vi "AlliGator Run XY Graph Python Function (API v1.1).vi"(6 "Mouse Click Event Data":T1, 7 "AlliGator Ctrl Refnums":T8, 8 "error in (no error)":errorcluster, 9 "data value reference in":refnum<data-value>, 10 "Python Function Info":T4, 11 "Python Session ID":refnum<k35>) -> (0 "error out":errorcluster, 1 "Data Value Reference out":refnum<data-value>, 2 "JSON String":string, 3 "Function Display Name":string, 4 "Function Parameters JSON String":string, 5 "Message":string)   [LabVIEW 2021, in "AlliGator Python Plugins.lvlib"]
uses:
  AlliGator Python Plugins.lvlib
  GUI/AlliGator Ctrl Refnums.ctl
  GUI/AlliGator Other Ctrl Refnums.ctl
  GUI/AlliGator State Indicator.ctl
  GUI/AlliGator Main Window Tabs.ctl
  GUI/AlliGator Phasor Plot Ctrl Refnums.ctl
  GUI/AlliGator Phasor Graph Ctrl Refnums.ctl
  Phasor/Phasor Calibration Type.ctl
  GUI/AlliGator Dataset Ctrl Refnums.ctl
  Source Image/AlliGator Displayed Image.ctl
  GUI/AlliGator Registered Events Ctrl Refnums.ctl
  GUI/AlliGator Image Histogram Control Refnums.ctl
  Histograms/Linear Histogram Options.ctl
  Histograms/Histogram Bin Option.ctl
  Histograms/Histogram Bin Position.ctl
  Decay Fit Parameter Map/AlliGator Decay Fit Map Control Refnums.ctl
  Fits/IRF(X)PSED/Decay Fit Parameters & Derived Quantities List v2.ctl
  Parameter Map/AlliGator Parameter Map Control Refnums.ctl
  Internal Variables/AlliGator Internal Variables v2.ctl
  <vilib>/vision/Image Controls.llb/IMAQ Image.ctl
  Internal Variables/AlliGator Gate Image Set.ctl
  Files/AlliGator FLI Dataset Type.ctl
  Files/AlliGator Data Series Type.ctl
  Dual-Channel Datasets/AlliGator Dataset Channel.ctl
  Settings/AlliGator Gate Arithmetic.ctl
  Image/Named ROI Description.ctl
  Phasor Graph/AlliGator Decay Metadata v3.ctl
  Decay Analysis/Decay Preprocessing/AlliGator Decay Background Subtraction Info.ctl
  Decay Analysis/Decay Preprocessing/AlliGator Baseline Subtraction Method.ctl
  Graphs/XY Graph/XY Graph Plot Shift Parameters.ctl
  Graphs/XY Graph/XY Graph Plot Shift Method.ctl
  Decay Analysis/Decay Preprocessing/AlliGator Decay Extrapolation Parameters.ctl
  Phasor/Calibration Phasor (m, phi).ctl
  Phasor/Phasor Reference Series.ctl
  Phasor/Phasor Calibration Map v2.ctl
  Phasor/Phasor (g, s).ctl
  Phasor Graph/AlliGator Raw Phasor Plot Data v5.ctl
  Phasor/Phasor Standard Deviation Options.ctl
  Phasor Plot/AlliGator Phasor Multi-Harmonic Data.ctl
  Phasor/Phasor Harmonic Data.ctl
  Decay Fit Parameter Map/AlliGator Decay Fit Options & Parameters v4.ctl
  Fits/IRF(X)PSED/Decay Fit Options v4.ctl
  Fits/Decay Convolution/Decay Model.ctl
  Fits/Residual Type.ctl
  Fits/IRF(X)PSED/Fit Weights Type v2.ctl
  Fits/Non-linear Fitting Method v2.ctl
  Fits/Fit Calculation Method.ctl
  Fits/Non-linear Fitting Algorithm.ctl
  Decay Analysis/Decay Fit/AlliGator Decay Fit Parameter Constraints 2.ctl
  Fits/IRF(X)PSED/Decay Fit Parameters In List.ctl
  Fits/IRF(X)PSED/MLE Baseline Offset Type.ctl
  Decay Analysis/Decay Preprocessing/AlliGator Decay Preprocessing Parameters.ctl
  Fits/IRF(X)PSED/Decay Fit Result Constraint.ctl
  Decay Fit Parameter Map/AlliGator Parameter Maps Data.ctl
  AlliGator Python Function Information.ctl
  AlliGator Python Function Parameter Definition.ctl
  AlliGator Python Function Output Definition.ctl
  AlliGator Python Plugin Target Type.ctl
  Graphs/XY Graph/XY Graph Mouse Click Event Data.ctl
  Graphs/XY Graph/XY Graph Refnum.ctl
  <vilib>/Utility/miscctls.llb/LVPoint32TypeDef.ctl
  API v1/AlliGator Python Plugin Plot Data v1.ctl
  API v1/AlliGator Python Plugin Graph Data v1.ctl
  AlliGator Python Plugin Data v1.1.ctl
  API v1/AlliGator Python Plugin Image Data v1.ctl
  AlliGator Python Plugin Parameter Map Data v1.1.ctl
  Image/Image Point.ctl
  AlliGator Python Plugin FLI Dataset Data v1.1.ctl
  Graphs/Get Plot at Mouse Click (XY Graph)/Get Plot at Mouse Click [AAC].vi
  Graphs/Graphs.lvlib
  Graphs/XY Graph/XY Graph Add-Ons.lvlib
  Strings/Strings.lvlib
  Error/Error.lvlib
  Image/Image.lvlib
  GUI/AlliGator GUI.lvlib
  Source Image/AlliGator Source Image.lvlib
  Phasor/Phasor.lvlib
  Histograms/Histogram Window.lvlib
  Fits/Fits.lvlib
  Decay Fit Parameter Map/AlliGator Decay Fit Parameter Map.lvlib
  Parameter Map/AlliGator Parameter Map.lvlib
  Decay Analysis/Decay Preprocessing/AlliGator Decay Preprocessing.lvlib
  Phasor Graph/AlliGator Phasor Graph.lvlib
  Files/AlliGator Files.lvlib
  Internal Variables/AlliGator Internal Variables.lvlib
  Phasor Plot/AlliGator Phasor Plot.lvlib
  Decay Analysis/Decay Fit/AlliGator Decay Fit.lvlib
  Settings/AlliGator Settings.lvlib
  Dual-Channel Datasets/AlliGator Dual-Channel Datasets.lvlib
panel:
  # "see the License on the block diagram (Ctrl+E or Window:Show Block Diagram)"
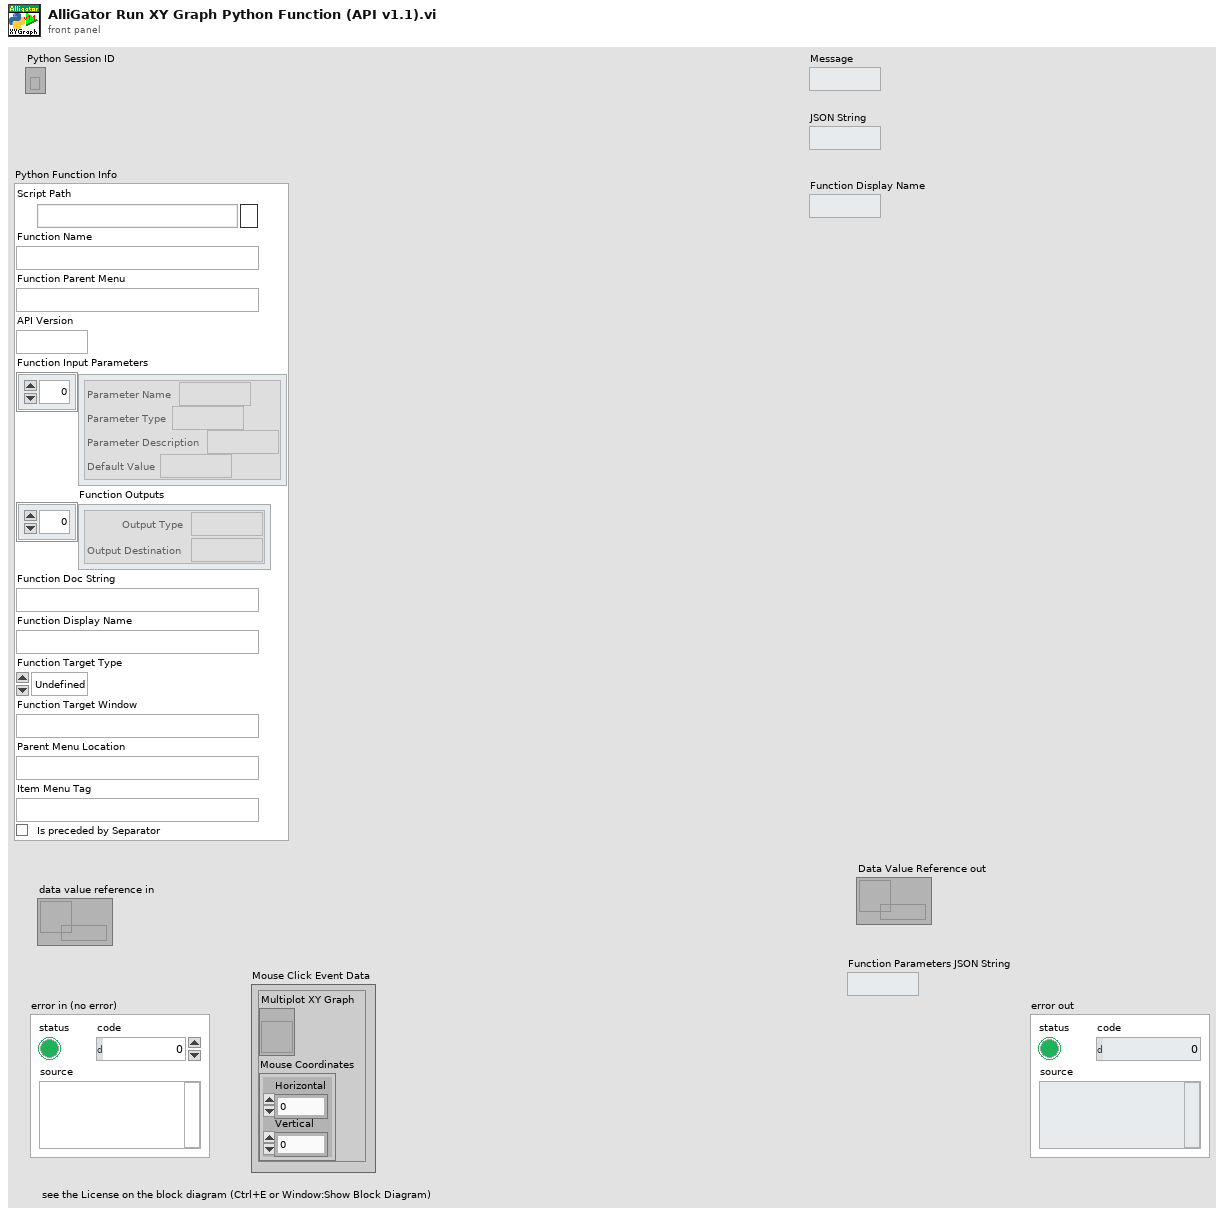
[diagram p1: front panel]
types:
  T1 = typedef "XY Graph Add-Ons.lvlib/XY Graph Mouse Click Event Data.ctl" = cluster{"Multiplot XY Graph":T2, "Mouse Coordinates":T3}
  T2 = typedef "XY Graph Add-Ons.lvlib/XY Graph Refnum.ctl" = refnum<vi>
  T3 = typedef "LVPoint32TypeDef.ctl" = cluster{"Horizontal":i32, "Vertical":i32}
  T4 = typedef "AlliGator Python Plugins.lvlib/AlliGator Python Function Information.ctl" = cluster{"Script Path":path, "Function Name":string, "Function Parent Menu":string, "API Version":string, "Function Input Parameters":T5[], "Function Outputs":T6[], "Function Doc String":string, "Function Display Name":string, "Function Target Type":T7, "Function Target Window":string, "Parent Menu Location":string, "Item Menu Tag":string, "Is preceded by Separator":bool}
  T5 = typedef "AlliGator Python Plugins.lvlib/AlliGator Python Function Parameter Definition.ctl" = cluster{"Parameter Name":string, "Parameter Type":string, "Parameter Description":string, "Default Value":string}
  T6 = typedef "AlliGator Python Plugins.lvlib/AlliGator Python Function Output Definition.ctl" = cluster{"Output Type":string, "Output Destination":string}
  T7 = typedef "AlliGator Python Plugins.lvlib/AlliGator Python Plugin Target Type.ctl" = enum16{"Undefined", "Window Menu", "Object Menu"}
  T8 = typedef "AlliGator GUI.lvlib/AlliGator Ctrl Refnums.ctl" = cluster{"Other AlliGator Ctrl Refnums":T9, "Phasor Plot Ctrl Refnums":T10, "Phasor Graph Ctrl Refnums":T11, "Dataset Control Refnums":T12, "Registered Events Ctrl Refnums":T13, "Image Histogram Ctrl Refnums":T14, "Decay Fit Map Ctrl Refnums":T15, "Parameter Map Ctrl Refnums":T16}
  T9 = typedef "AlliGator GUI.lvlib/AlliGator Other Ctrl Refnums.ctl" = cluster{"State Indicators":refnum<vi>, " Progress Bar":refnum<vi>, "Decay Graph Active":refnum<vi>, "Decay Statistics Bin":refnum<vi>, "Time Step":refnum<vi>, "Use File Timestamp":refnum<vi>, "Tab Control":refnum<vi>, "CPU":refnum<vi>, "Abort Fit":refnum<vi>, "Dataset File/Folder Path":refnum<vi>, "Abort ROI Creation":refnum<vi>, "Event LED":refnum<vi>, "Dataset File/Folder Path 2":refnum<vi>, "Dataset File/Folder Path 3":refnum<vi>, "Dataset File/Folder Path 4":refnum<vi>, "Dataset File/Folder Path 5":refnum<vi>, "Dataset File/Folder Path 6":refnum<vi>, "Dataset File/Folder Path 7":refnum<vi>, "Dataset File/Folder Path 8":refnum<vi>, "Dataset File/Folder Path 9":refnum<vi>, "Dataset File/Folder Path 10":refnum<vi>, "Dataset File/Folder Path 11":refnum<vi>}
  T10 = typedef "AlliGator GUI.lvlib/AlliGator Phasor Plot Ctrl Refnums.ctl" = cluster{"Phasor Ratio":refnum<vi>, "Modulus Lifetime":refnum<vi>, "Phasor at cursor (m, phi)":refnum<vi>, "Phase Lifetime":refnum<vi>, "Phasor at cursor (g, s)":refnum<vi>, "Phasor Plor Average Lifetime":refnum<vi>, "Phasor Plot Active":refnum<vi>, "Save Phasor Plot":refnum<vi>, "Image Overlay Color":refnum<vi>, "Phasor Plot Color Scale":refnum<vi>, "Reference 1 Button":refnum<vi>, "Reference 2 Button":refnum<vi>, "True Phasor Plot Value":refnum<vi>}
  T11 = typedef "AlliGator GUI.lvlib/AlliGator Phasor Graph Ctrl Refnums.ctl" = cluster{"Phasor Ratio":refnum<vi>, "Modulus Lifetime":refnum<vi>, "Phasor at cursor (m, phi)":refnum<vi>, "Phase Lifetime":refnum<vi>, "Phasor at cursor (g, s)":refnum<vi>, "Phasor Graph Average Lifetime":refnum<vi>, "Phasor Graph Active":refnum<vi>, "Save Phasor Graph":refnum<vi>, "Phasor Frame Slide":refnum<vi>, "Single Step Phasor":refnum<vi>, "Calibration Type":refnum<vi>, "Show Line":refnum<vi>, "Phase Lifetime 1":refnum<vi>, "Phase Lifetime 2":refnum<vi>, "Phasor Graph Frequency":refnum<vi>, "Phasor Reference 1 Control":refnum<vi>, "Phasor Reference 2 Control":refnum<vi>, "Calibration Lifetime":refnum<vi>, "Phase Lifetime SDV":refnum<vi>, "Average Lifetime SDV":refnum<vi>, "Phasor Ratio SDV":refnum<vi>, "Modulus Lifetime SDV":refnum<vi>}
  T12 = typedef "AlliGator GUI.lvlib/AlliGator Dataset Ctrl Refnums.ctl" = cluster{"Current Data":refnum<vi>, "Gate Image Slide":refnum<vi>, "Time Point Slide":refnum<vi>, "Current Time Stamp":refnum<vi>, "Save Image":refnum<vi>, "Displayed Image":refnum<vi>, "Overlay Mode":refnum<vi>, "Phasor Overlay Color":refnum<vi>, "Image Color Scale":refnum<vi>, "Use ROI as Search Area":refnum<vi>, "Source Image ROI Color":refnum<vi>, "True Pixel Value":refnum<vi>}
  T13 = typedef "AlliGator GUI.lvlib/AlliGator Registered Events Ctrl Refnums.ctl" = cluster{"Time Point Slider":refnum<vi>, "Phasor Plot Display Range":refnum<vi>, "Decay Graph":refnum<vi>, "Decay Statistics Graph":refnum<vi>, "Intensity Time Trace":refnum<vi>, "Phasor Graph":refnum<vi>, "Phasor Ratio Graph":refnum<vi>, "Lifetime Graph":refnum<vi>, "Phasor Plot Display":refnum<vi>, "Source Image Display":refnum<vi>, "Decay Fit Parameter Map Display Range":refnum<vi>, "Decay Fit Parameter Map Display":refnum<vi>, "Parameter Map Display Range":refnum<vi>, "Parameter Map Display":refnum<vi>, "Phasor Plot Display Range":refnum<vi>}
  T14 = typedef "AlliGator GUI.lvlib/AlliGator Image Histogram Control Refnums.ctl" = cluster{"Image Histogram":refnum<vi>, "Image Histogram Options":refnum<vi>, "Image Histogram Active":refnum<vi>, "Image Histogram Upper Percentile":refnum<vi>, "Image Histogram Lower Percentile":refnum<vi>, "Auto-Adjust Contrast":refnum<vi>}
  T15 = typedef "AlliGator Decay Fit Parameter Map.lvlib/AlliGator Decay Fit Map Control Refnums.ctl" = cluster{"Decay Fit Parameter Map Color Scale":refnum<vi>, "Decay Fit Parameter":refnum<vi>, "Max Parameter":refnum<vi>, "Min Parameter":refnum<vi>, "Decay Fit Parameter Map Display":refnum<vi>, "Decay Fit Parameter Map Display Range":refnum<vi>, "Decay Parameter Map X":refnum<vi>, "Decay Parameter Map Y":refnum<vi>, "Decay Parameter Map Value":refnum<vi>}
  T16 = typedef "AlliGator Parameter Map.lvlib/AlliGator Parameter Map Control Refnums.ctl" = cluster{"Parameter Map Color Scale":refnum<vi>, "Map Parameter":refnum<vi>, "Max Parameter":refnum<vi>, "Min Parameter":refnum<vi>, "Parameter Map Display":refnum<vi>, "Parameter Map Display Range":refnum<vi>, "Parameter Map Set":refnum<vi>, "Parameter Map X":refnum<vi>, "Parameter Map Y":refnum<vi>, "Parameter Map Value":refnum<vi>}
  T17 = typedef "AlliGator Python Plugins.lvlib/AlliGator Python Plugin Data v1.1.ctl" = cluster{"Image_Plugin_Data":T18, "Graph_Plugin_Data":T19, "Parameter_Map_Plugin_Data":T21, "FLI_Dataset_Plugin_Data":T23}
  T18 = typedef "AlliGator Python Plugins.lvlib/AlliGator Python Plugin Image Data v1.ctl" = cluster{"Image_Name":string, "Image":sgl[][]}
  T19 = typedef "AlliGator Python Plugins.lvlib/AlliGator Python Plugin Graph Data v1.ctl" = cluster{"Graph_Name":string, "Plots":T20[], "Reference_Decay":T20}
  T20 = typedef "AlliGator Python Plugins.lvlib/AlliGator Python Plugin Plot Data v1.ctl" = cluster{"Plot_Name":string, "X_Array":dbl[], "Y_Array":dbl[]}
  T21 = typedef "AlliGator Python Plugins.lvlib/AlliGator Python Plugin Parameter Map Data v1.1.ctl" = cluster{"Parameter_Names":string[], "Parameter_Flattened_Map":dbl[][], "Locations":T22[], "IRF_X":dbl[], "IRF_Y_Flattened_List":dbl[][], "X_Resolution":i32, "Y_Resolution":i32}
  T22 = typedef "Image.lvlib/Image Point.ctl" = cluster{"X":i32, "Y":i32}
  T23 = typedef "AlliGator Python Plugins.lvlib/AlliGator Python Plugin FLI Dataset Data v1.1.ctl" = cluster{"FLI_Dataset_Name":string, "Gate_Duration":dbl, "Gate_Separation":dbl, "Gate_Number":i32, "X_Size":i32, "Y_Size":i32, "Image_Data_List":T18[], "Mask_Image":u16[][], "Sum_Image":sgl[][], "Max_Image":sgl[][], "Min_Image":sgl[][]}
  T24 = typedef "AlliGator Python Plugins.lvlib/AlliGator Type of Plot Data.ctl" = enum16{"Single Plot", "Selected Plots", "All Plots"}
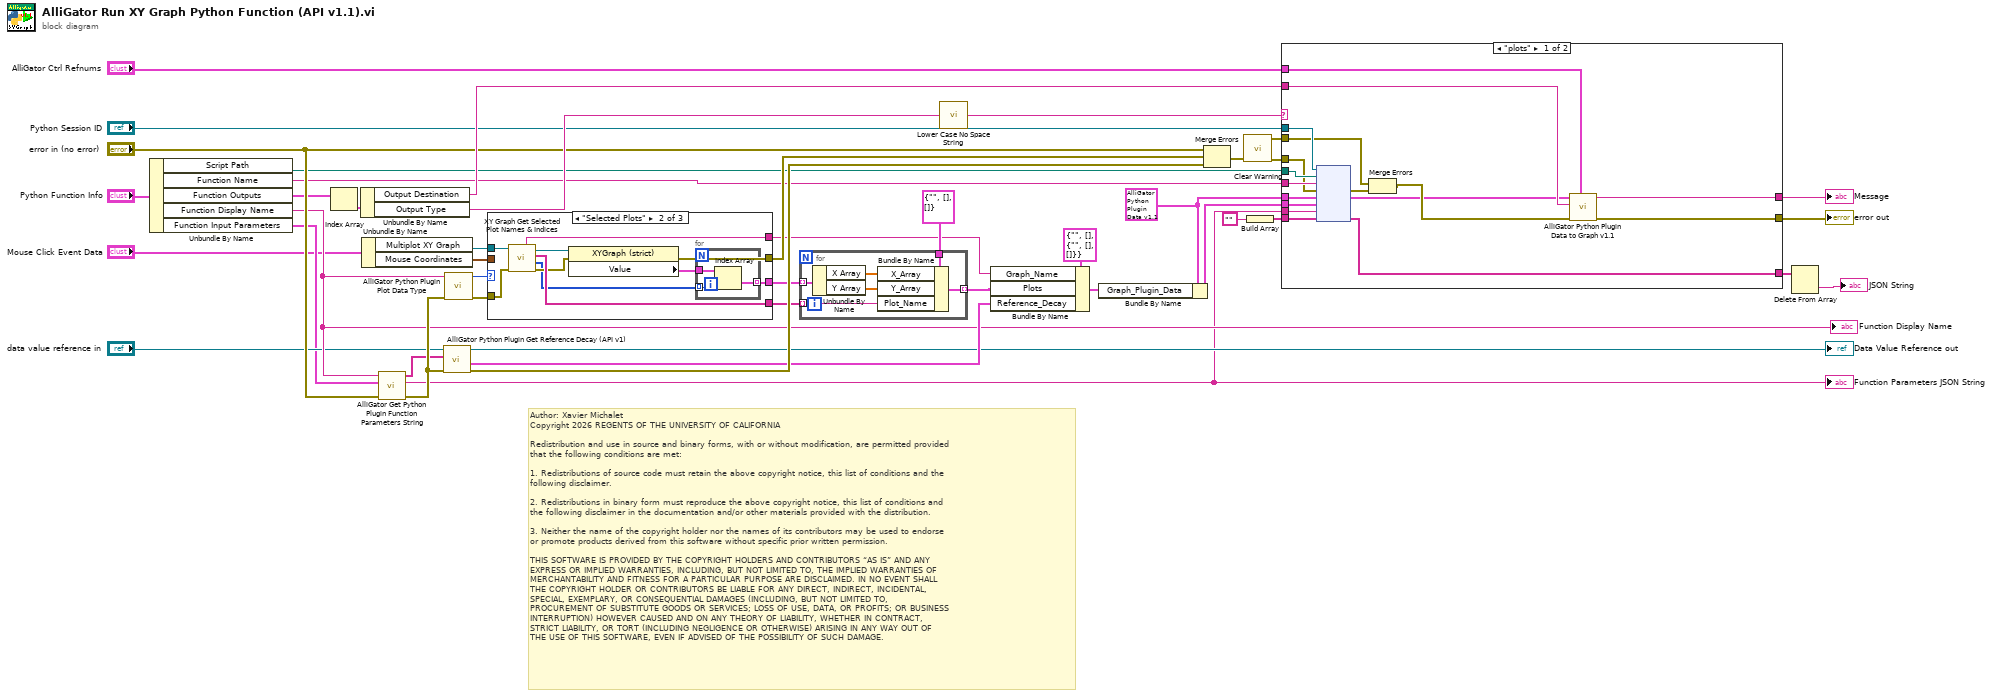
[diagram p0: block diagram]
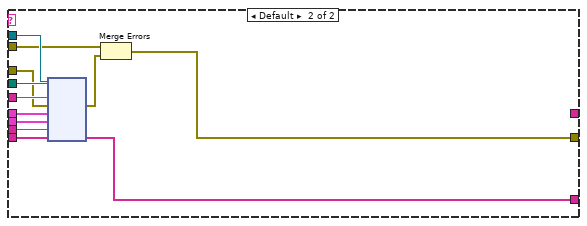
[diagram p2: hidden frame]
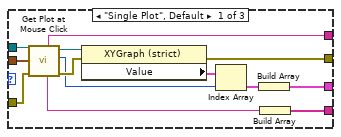
[diagram p3: hidden frame]
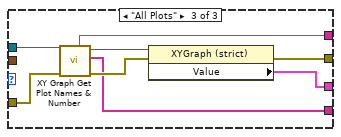
[diagram p4: hidden frame]
diagram:
  w1 = T17 {"Image_Plugin_Data"={"Image_Name"="", "Image"=[]}, "Graph_Plugin_Data"={"Graph_Name"="", "Plots"=[], "Reference_Decay"={"Plot_Name"="", "X_Array"=[], "Y_Array"=[]}}, "Parameter_Map_Plugin_Data"={"Parameter_Names"=[], "Parameter_Flattened_Map"=[], "Locations"=[], "IRF_X"=[], "IRF_Y_Flattened_List"=[], "X_Resolution"=0, "Y_Resolution"=0}, "FLI_Dataset_Plugin_Data"={"FLI_Dataset_Name"="", "Gate_Duration"=0.0, "Gate_Separation"=0.0, "Gate_Number"=0, "X_Size"=0, "Y_Size"=0, "Image_Data_List"=[], "Mask_Image"=[], "Sum_Image"=[], "Max_Image"=[], "Min_Image"=[]}} ("Plugin_Data")
  # "Author: Xavier Michalet\nCopyright 2026 REGENTS OF THE UNIVERSITY OF CALIFORNIA\n\nRedistribution and use in source and binary forms, with or without modification, are permitted provided\nthat the following conditions are met:\n\n1. Redistributions of source code must retain the above copyright notice, this list of conditions and the\nfollowing disclaimer.\n\n2. Redistributions in binary form must reproduce the above copyright notice, this list of conditions and\nthe following disclaimer in the documentation and/or other materials provided with the distribution.\n\n3. Neither the name of the copyright holder nor the names of its contributors may be used to endorse \nor promote products derived from this software without specific prior written permission.\n\nTHIS SOFTWARE IS PROVIDED BY THE COPYRIGHT HOLDERS AND CONTRIBUTORS “AS IS” AND ANY \nEXPRESS OR IMPLIED WARRANTIES, INCLUDING, BUT NOT LIMITED TO, THE IMPLIED WARRANTIES OF\nMERCHANTABILITY AND FITNESS FOR A PARTICULAR PURPOSE ARE DISCLAIMED. IN NO EVENT SHALL\nTHE COPYRIGHT HOLDER OR CONTRIBUTORS BE LIABLE FOR ANY DIRECT, INDIRECT, INCIDENTAL, \nSPECIAL, EXEMPLARY, OR CONSEQUENTIAL DAMAGES (INCLUDING, BUT NOT LIMITED TO, \nPROCUREMENT OF SUBSTITUTE GOODS OR SERVICES; LOSS OF USE, DATA, OR PROFITS; OR BUSINESS\nINTERRUPTION) HOWEVER CAUSED AND ON ANY THEORY OF LIABILITY, WHETHER IN CONTRACT, \nSTRICT LIABILITY, OR TORT (INCLUDING NEGLIGENCE OR OTHERWISE) ARISING IN ANY WAY OUT OF\nTHE USE OF THIS SOFTWARE, EVEN IF ADVISED OF THE POSSIBILITY OF SUCH DAMAGE."
  n1 = Unbundle By Name("Python Function Info") -> ("Script Path"=w9:path, "Function Name"=w12:string, "Function Outputs"=w15:T6[], "Function Display Name"=w14:string, "Function Input Parameters"=w10:T5[])
  "Function Display Name" <- w14
  n2 = Index Array(array=w15) -> (element=w39:T6)  [unwired: 1 in]
  n3 = Unbundle By Name(w39) -> ("Output Destination"=w42:string, "Output Type"=w40:string)
  n4 = Unbundle By Name("Mouse Click Event Data") -> ("Multiplot XY Graph"=w21:T2, "Mouse Coordinates"=w22:T3)
  n5 = call "AlliGator Get Python Plugin Function Parameters String.vi"("error in (no error)"="error in (no error)", "Function Parameters"=w10, "Function Display Name"=w14) -> ("error out"=w30:errorcluster, "Function Parameters JSON String"=w7:string, "Parameter Names Not Found"=w29:string[])  [unwired: 6 in]
  "Function Parameters JSON String" <- w7
  n6 = call "AlliGator Python Plugin Get Reference Decay (API v1).vi"("error in (no error)"=w30, "AlliGator Parameter Names in"=w29, "Data Value Reference in"="data value reference in") -> ("error out"=w44:errorcluster, "Reference Decay"=w31:T20, "Data Value Reference out"=→"Data Value Reference out":refnum<data-value>)  [unwired: 4 in, 2 out]
  n7 = call "AlliGator Python Plugin Plot Data Type.vi"("error in (no error)"=w30, "Function Name"=w14) -> ("error out"=w24:errorcluster, "Type of Plot Data"=w23:T24)  [unwired: 8 in]
  n8 = case shown="\"Selected Plots\"" w23 {
    tunnel: w21 -> [w53 w67 w76]
    tunnel: w22 -> [w52 _ _]
    tunnel: [w51 w58 w77] -> w43
    tunnel: [w48 w64 w71] -> w27
    tunnel: w24 -> [w49 w66 w75]
    tunnel: [w47 w59 w78] -> w26
    tunnel: [w46 w65 w72] -> w25
    frame "Single Plot", Default {
      n9 = call-poly "Get Plot at Mouse Click.vi"("error in (no error)"=w49, "Mouse Click Coordinates"=w52, "XY Graph in"=w53) -> ("error out"=w56:errorcluster, "Plot at Coordinates"=w54:i32, "XY Graph out"=w57:T2, "Plot Name"=w50:string, "Graph Name"=w46:string)  [unwired: 2 in, 2 out]
      n10 = property class="XYGraph (strict)"(reference=w57, error in=w56) -> (error out=w51:errorcluster, "Value"=w55:cluster{"X Array":dbl[], "Y Array":dbl[]}[])  [unwired: 1 out]
      n11 = Index Array(array=w55, index=w54) -> (element=w45:cluster{"X Array":dbl[], "Y Array":dbl[]})
      n12 = Build Array(w45) -> (w47:cluster{"X Array":dbl[], "Y Array":dbl[]}[])
      n13 = Build Array(w50) -> (w48:string[])
    }
    frame "Selected Plots" {
      n14 = call "XY Graph Get Selected Plot Names & Indices.vi"("error in (no error)"=w66, "XY Graph in"=w67) -> ("error out"=w63:errorcluster, "Selected Plot Indices"=w61:i32[], "Selected Plot Names"=w64:string[], "XY Graph out"=w62:T2, "Graph Name"=w65:string)  [unwired: 5 in]
      n15 = property class="XYGraph (strict)"(reference=w62, error in=w63) -> (error out=w58:errorcluster, "Value"=w60:cluster{"X Array":dbl[], "Y Array":dbl[]}[])  [unwired: 1 out]
      n16 = for {
        tunnel: w61 -> [w70] mode=indexing
        tunnel: w60 -> [w69]
        tunnel: [w68] -> w59 mode=indexing
        n17 = Index Array(array=w69, index=w70) -> (element=w68:cluster{"X Array":dbl[], "Y Array":dbl[]})
      }
    }
    frame "All Plots" {
      n18 = call "XY Graph Get Plot Names & Number.vi"("error in (no error)"=w75, "XYGraph in"=w76) -> ("error out"=w74:errorcluster, "Plot Names"=w71:string[], "XYGraph out"=w73:T2, "Graph Name"=w72:string)  [unwired: 4 in, 2 out]
      n19 = property class="XYGraph (strict)"(reference=w73, error in=w74) -> (error out=w77:errorcluster, "Value"=w78:cluster{"X Array":dbl[], "Y Array":dbl[]}[])  [unwired: 1 out]
    }
  }
  n20 = for {
    tunnel: w27 -> [w84] mode=indexing
    tunnel: [w83] -> w32 mode=indexing
    tunnel: w26 -> [w82] mode=indexing
    tunnel: T20 {"Plot_Name"="", "X_Array"=[], "Y_Array"=[]} ("Plugin Plot Data") -> [w79]
    n21 = Unbundle By Name(w82) -> ("X Array"=w81:dbl[], "Y Array"=w80:dbl[])
    n22 = Bundle By Name(cluster=w79, "X_Array"=w81, "Y_Array"=w80, "Plot_Name"=w84) -> (w83:T20)
  }
  n23 = call "Lower Case No Space String.vi"("String"=w40) -> ("Lower Case No Space String"=w41:string)
  n24 = Bundle By Name(cluster=T19 {"Graph_Name"="", "Plots"=[], "Reference_Decay"={"Plot_Name"="", "X_Array"=[], "Y_Array"=[]}} ("Graph Plugin Data"), "Graph_Name"=w25, "Plots"=w32, "Reference_Decay"=w31) -> (w3:T19)
  n25 = Bundle By Name(cluster=w1, "Graph_Plugin_Data"=w3) -> (w4:T17)
  n26 = Merge Errors("error in (no error)", w43, w44) -> (w36:errorcluster)
  n27 = call "Clear Warning.vi"("error in (no error)"=w36) -> ("cleared warning or error dup"=w37:errorcluster, "error in (dup)"=w38:errorcluster)  [unwired: 9 in]
  n28 = Build Array("") -> (w35:string[])
  n29 = case shown="\"plots\"" w41 {
    tunnel: "Python Session ID" -> [w101 w113]
    tunnel: w7 -> [w100 w112]
    tunnel: w9 -> [w99 w111]
    tunnel: [w98 w110] -> w28
    tunnel: w12 -> [w96 w108]
    tunnel: w4 -> [w95 w107]
    tunnel: w1 -> [w94 w106]
    tunnel: w35 -> [w93 w105]
    tunnel: w37 -> [w92 w104]
    tunnel: w38 -> [w91 w103]
    tunnel: [w90 _] -> w16
    tunnel: [w89 w102] -> w17
    tunnel: w42 -> [w87 _]
    tunnel: "AlliGator Ctrl Refnums" -> [w86 _]
    frame "plots" {
      n30 = node(w101, w99, w96, w92, w94, w95, w100, w93) -> (w97:errorcluster, w85:T17, w98:string[])  [unwired: 2 in, 3 out]
      n31 = Merge Errors(w91, w97) -> (w88:errorcluster)
      n32 = call "AlliGator Python Plugin Data to Graph v1.1.vi"("AlliGator Ctrl Refnums"=w86, "error in (no error)"=w88, "Output Destination"=w87, "Plugin_Data"=w85) -> ("error out"=w89:errorcluster, "Message"=w90:string)  [unwired: 6 in]
    }
    frame Default {
      n33 = node(w113, w111, w108, w104, w106, w107, w112, w105) -> (w109:errorcluster, w110:string[])  [unwired: 3 in, 3 out]
      n34 = Merge Errors(w103, w109) -> (w102:errorcluster)
    }
  }
  "error out" <- w17
  "Message" <- w16
  n35 = Delete From Array(array=w28) -> (deleted portion=→"JSON String":string)  [unwired: 2 in, 1 out]
